vi "Save Object as VI.vi"(8 "error in (no error)":errorcluster, 9 "Name":string, 11 "Object in":refnum<vi>) -> (0 "error out":errorcluster, 3 "Object out":refnum<vi>, 5 "Ok?":bool)   [LabVIEW 2024]
uses:
  <vilib>/Utility/miscctls.llb/LVPositionTypeDef.ctl
  <vilib>/Utility/NIReport.llb/NI_ReportGenerationCore.lvlib
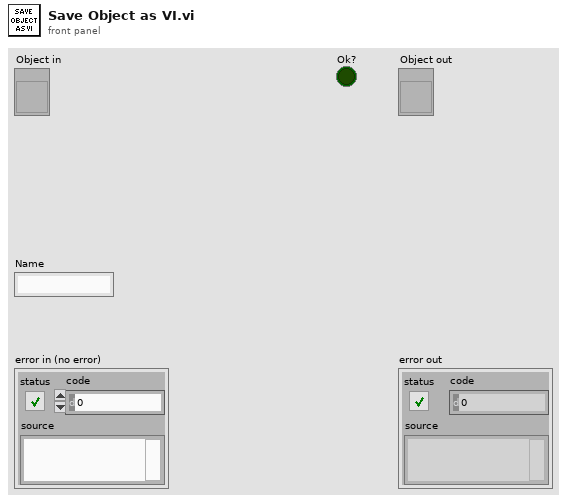
[diagram p1: front panel]
types:
  T1 = typedef "LVPositionTypeDef.ctl" = cluster{"Left":i32, "Top":i32}
  T2 = typedef "imagedata.ctl" = cluster{"image type":i32, "image depth":i32, "image":u8[], "mask":u8[], "colors":u32[], "Rectangle":cluster{"left":i16, "top":i16, "right":i16, "bottom":i16}}
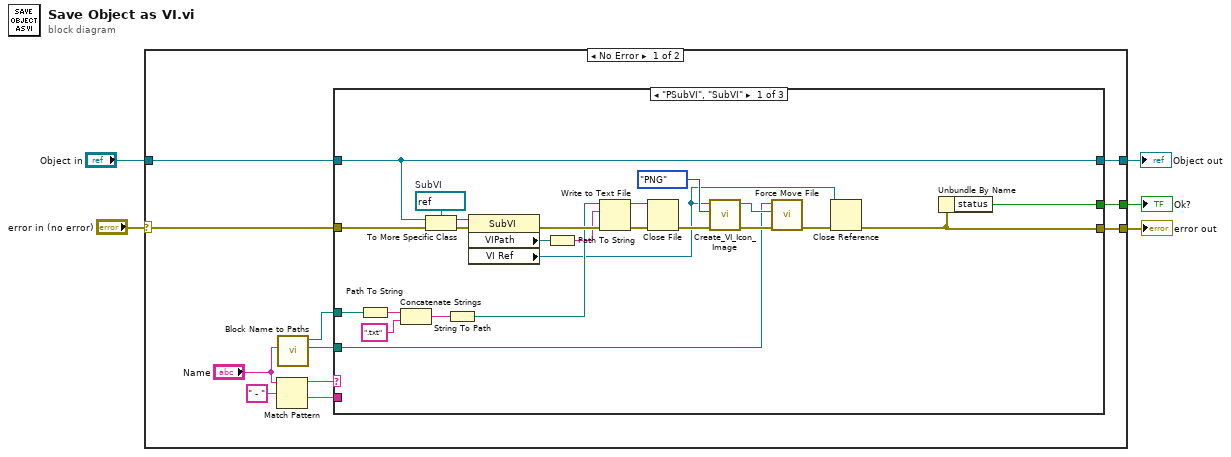
[diagram p0: block diagram]
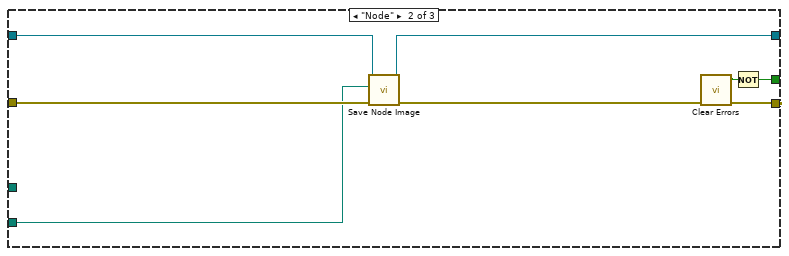
[diagram p2: hidden frame]
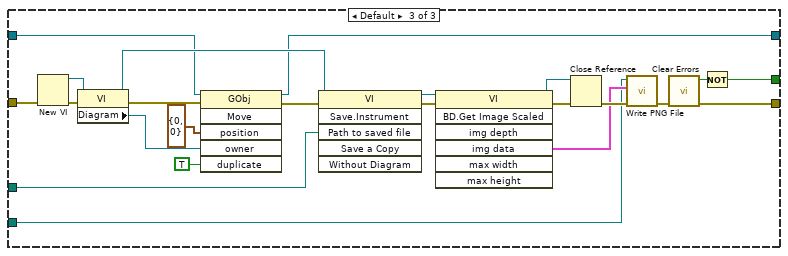
[diagram p3: hidden frame]
diagram:
  n1 = case shown="No Error" "error in (no error)" {
    selector: "error in (no error)" -> [w16 w74]
    tunnel: [w15 w74] -> w5
    tunnel: [w14 FALSE ("specific error cleared?")] -> w3
    tunnel: [w8 w72] -> w2
    tunnel: "Object in" -> [w7 w72]
    frame No Error {
      n2 = Match Pattern(string="Name", regular expression=" - ") -> (before substring=w12:string, after substring=w6:string)  [unwired: 1 in, 2 out]
      n3 = call "Block Name to Paths.vi"("Block Name"="Name") -> ("Image Path"=w9:path, "Block Path"=w10:path)  [unwired: 9 in]
      n4 = case shown="\"PSubVI\", \"SubVI\"" w12 {
        tunnel: w16 -> [w37 w45 w57]
        tunnel: [w18 w47 w55] -> w15
        tunnel: [w20 w46 w53] -> w14
        tunnel: w10 -> [w36 _ w52]
        tunnel: w9 -> [w22 w41 w51]
        tunnel: w7 -> [w21 w43 w50]
        tunnel: [w21 w42 w49] -> w8
        tunnel: w6 -> [_ _ _]
        frame "PSubVI", "SubVI" {
          w40 = refnum<vi> refnum  # SubVI
          n5 = Path To String(path=w36) -> (string=w35:string)
          n6 = Concatenate Strings(w35, ".txt" ("string")) -> (w32:string)
          n7 = To More Specific Class(target class=w40, reference=w21, error in=w37) -> (specific class reference=w38:refnum<vi>, error out=w39:errorcluster)
          n8 = String To Path(string=w32) -> (path=w31:path)
          n9 = property on="Property Node" class="SubVI"(reference=w38, error in=w39) -> (error out=w33:errorcluster, "VIPath"=w30:path, "VI Ref"=w17:refnum<vi>)  [unwired: 1 out]
          n10 = Path To String(path=w30) -> (string=w29:string)
          n11 = Write to Text File(file (use dialog)=w31, text=w29, error in=w33) -> (refnum out=w27:refnum<file>, error out=w28:errorcluster)  [unwired: 1 in, 1 out]
          n12 = Close File(refnum=w27, error in=w28) -> (error out=w26:errorcluster)  [unwired: 1 out]
          n13 = call <vilib>:"Create_VI_Icon_Image.vi"("error in (no error)"=w26, "Image Format (jpeg)"=enum32{"PNG", "JPEG", "GIF"}."PNG", "VI"=w17) -> ("error out"=w24:errorcluster, "Path to image"=w23:path)  [unwired: 7 in]
          n14 = call "Force Move File.vi"("error in"=w24, "Source Path"=w23, "Target Path in"=w22) -> ("error out"=w19:errorcluster)  [unwired: 7 in, 1 out]
          n15 = Close Reference(reference=w17, error in (no error)=w19) -> (error out=w18:errorcluster)
          n16 = Unbundle By Name(w18) -> ("status"=w20:bool)
        }
        frame "Node" {
          n17 = call "Save Node Image.vi"("error in (no error)"=w45, "Image Path"=w41, "Object in"=w43) -> ("error out"=w44:errorcluster, "Object out"=w42:refnum<vi>)  [unwired: 7 in]
          n18 = call <vilib>:"Clear Errors.vi"("error in (no error)"=w44) -> ("error out"=w47:errorcluster, "specific error cleared?"=w48:bool)  [unwired: 5 in]
          n19 = Not(x=w48) -> (.not. x?=w46:bool)
        }
        frame Default {
          n20 = New VI(8:w57) -> (0:w70:errorcluster, 3:w71:refnum<vi>)  [unwired: 6 in]
          n21 = property class="VI"(reference=w71, error in=w70) -> (reference out=w66:refnum<vi>, error out=w60:errorcluster, "Diagram"=w67:refnum<vi>)
          n22 = invoke class="GObj" method="Move"(reference=w50, error in=w60, "position"=T1 {"Left"=0, "Top"=0}, "owner"=w67, "duplicate"=TRUE ("Duplicate? (F)")) -> (reference out=w49:refnum<vi>, error out=w65:errorcluster)  [unwired: 1 in, 4 out]
          n23 = invoke class="VI" method="Save.Instrument"(reference=w66, error in=w65, "Path to saved file"=w52) -> (reference out=w64:refnum<vi>, error out=w62:errorcluster)  [unwired: 3 in, 4 out]
          n24 = invoke class="VI" method="BD.Get Image Scaled"(reference=w64, error in=w62) -> (reference out=w63:refnum<vi>, error out=w61:errorcluster, "img data"=w58:T2)  [unwired: 5 in, 4 out]
          n25 = Close Reference(reference=w63, error in (no error)=w61) -> (error out=w59:errorcluster)
          n26 = call <vilib>:"Write PNG File.vi"("error in (no error)"=w59, "image data"=w58, "path to PNG file"=w51) -> ("error out"=w56:errorcluster)  [unwired: 7 in, 1 out]
          n27 = call <vilib>:"Clear Errors.vi"("error in (no error)"=w56) -> ("error out"=w55:errorcluster, "specific error cleared?"=w54:bool)  [unwired: 5 in]
          n28 = Not(x=w54) -> (.not. x?=w53:bool)
        }
      }
    }
    frame Error {
    }
  }
  "error out" <- w5
  "Ok?" <- w3
  "Object out" <- w2
